vi "Facade.vi"(0 "Data In":T5, 2 "Display State In":T3, 3 "Container State":T4) -> (6 "Data Out":T5, 7 "Display State Out":T3, 8 "Action":T2)   [LabVIEW 2014, in "Mux XControl.xctl"]
uses:
  Mux XControl.xctl
  <vilib>/_xctls/Action.ctl
  <vilib>/_xctls/XControlSupport.lvlib
  <vilib>/_xctls/Container State.ctl
  Data.ctl
  State.ctl
  ChannelType.ctl
panel:
  in  "Channels":T1
  in  "path to image file":path
  out "CtlBckgrnd":picture
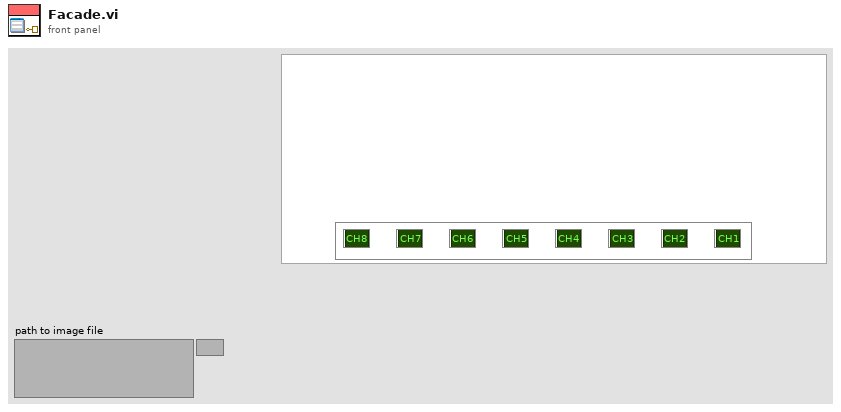
[diagram p1: front panel]
types:
  T1 = cluster{"Ch1":cluster{"StartPoint":cluster{"x":i16, "y":i16}, "RailPoint1":cluster{"x":i16, "y":i16}, "Ch1":bool}, "Ch2":cluster{"StartPoint":cluster{"x":i16, "y":i16}, "RailPoint1":cluster{"x":i16, "y":i16}, "Ch1":bool}, "Ch3":cluster{"StartPoint":cluster{"x":i16, "y":i16}, "RailPoint1":cluster{"x":i16, "y":i16}, "Ch1":bool}, "Ch4":cluster{"StartPoint":cluster{"x":i16, "y":i16}, "RailPoint1":cluster{"x":i16, "y":i16}, "Ch1":bool}, "Ch5":cluster{"StartPoint":cluster{"x":i16, "y":i16}, "RailPoint1":cluster{"x":i16, "y":i16}, "Ch1":bool}, "Ch6":cluster{"StartPoint":cluster{"x":i16, "y":i16}, "RailPoint1":cluster{"x":i16, "y":i16}, "Ch1":bool}, "Ch7":cluster{"StartPoint":cluster{"x":i16, "y":i16}, "RailPoint1":cluster{"x":i16, "y":i16}, "Ch1":bool}, "Ch8":cluster{"StartPoint":cluster{"x":i16, "y":i16}, "RailPoint1":cluster{"x":i16, "y":i16}, "Ch1":bool}}
  T2 = typedef "XControlSupport.lvlib/Action.ctl" = cluster{"Data Changed?":bool, "State Changed?":bool, "Action Name":string}
  T3 = typedef "Mux XControl.xctl/State.ctl" = cluster{"Numeric":dbl}
  T4 = typedef "XControlSupport.lvlib/Container State.ctl" = cluster{"Indicator?":bool, "Run Mode?":bool, " Refnum":refnum<vi>}
  T5 = typedef "Mux XControl.xctl/Data.ctl" = cluster{"From Ch":T6, "Into Ch":T6}
  T6 = typedef "Mux XControl.xctl/ChannelType.ctl" = enum16{"Ch1", "Ch2", "Ch3", "Ch4", "Ch5", "Ch6", "Ch7", "Ch8", "MuxOut"}
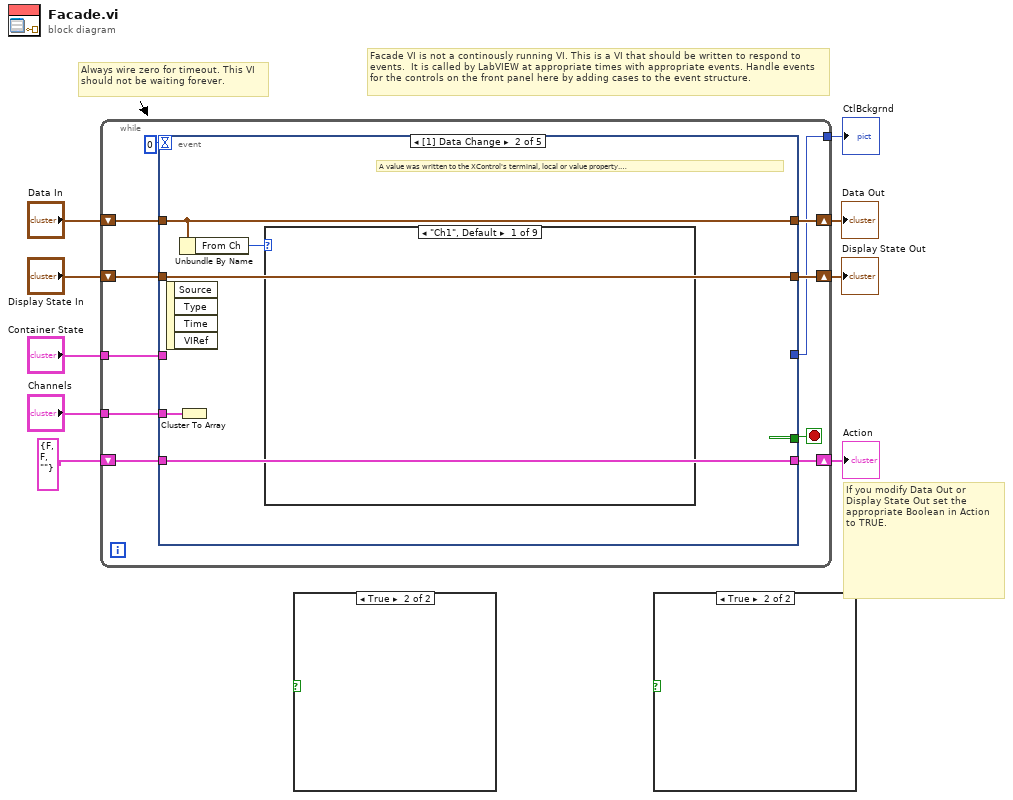
[diagram p0: block diagram]
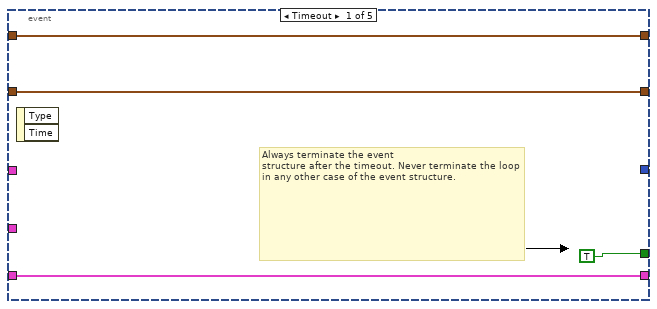
[diagram p4: hidden frame]
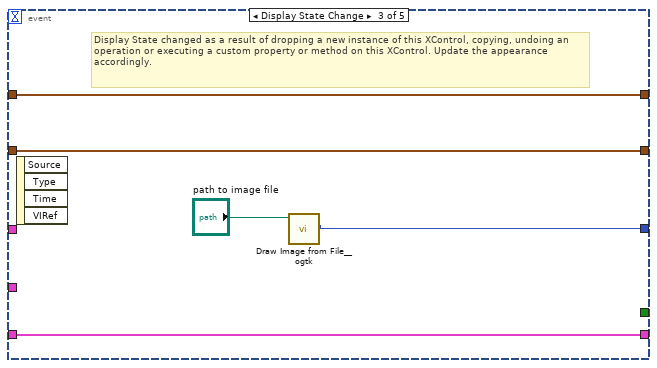
[diagram p13: hidden frame]
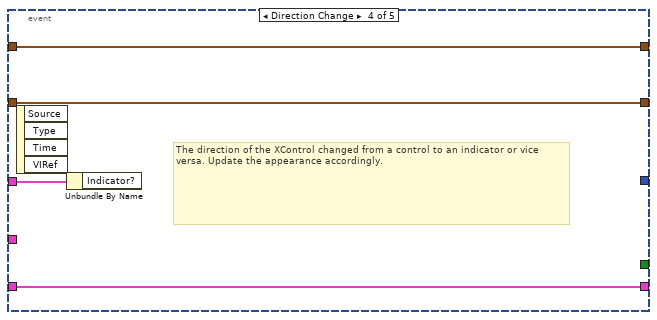
[diagram p14: hidden frame]
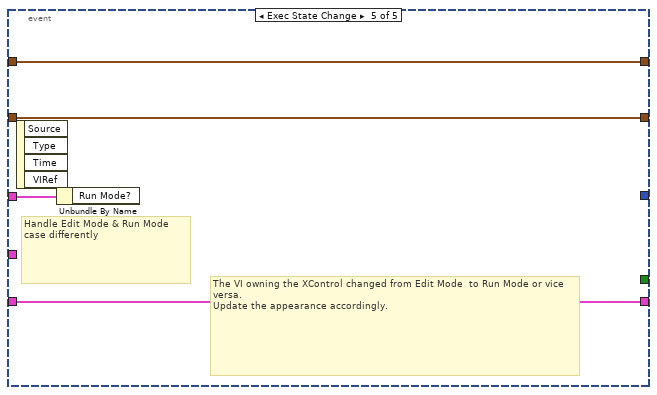
[diagram p15: hidden frame]
diagram:
  # "Always wire zero for timeout. This VI should not be waiting forever."
  # "Facade VI is not a continously running VI. This is a VI that should be written to respond to events.  It is called by LabVIEW at appropriate times with appropriate events. Handle events for the controls on the front panel here by adding cases to the event structure."
  # "If you modify Data Out or\nDisplay State Out set the\nappropriate Boolean in Action\nto TRUE."
  n1 = while {
    shift-right: [w19] -> w6
    shift-left: "Display State In" -> [w20]
    tunnel: "Container State" -> [w16]
    shift-right: [w14] -> w9
    shift-left: "Data In" -> [w15]
    shift-right: [w12] -> w4
    shift-left: T2 {"Data Changed?"=FALSE, "State Changed?"=FALSE, "Action Name"=""} ("Action") -> [w13]
    tunnel: "Channels" -> [w11]
    tunnel: [w10] -> w1
    stop <- w18 stop-if-true
    n2 = event shown="[1] Data Change" {
      selector: _ -> [_ _ _ _ _]
      dyn-events: _ -> [_ _ _ _ _]
      timeout: 0 -> [_ _ _ _ _]
      tunnel: w20 -> [w22 w29 w34 w37 w41]
      tunnel: [w22 w29 w34 w37 w41] -> w19
      tunnel: [TRUE _ _ _ _] -> w18
      tunnel: w16 -> [_ _ _ w38 w42]
      tunnel: w15 -> [w21 w27 w33 w36 w40]
      tunnel: [w21 w27 w33 w36 w40] -> w14
      tunnel: [w23 w28 w32 w35 w39] -> w12
      tunnel: w13 -> [w23 w28 w32 w35 w39]
      tunnel: w11 -> [_ w26 _ _ _]
      tunnel: [_ _ w30 _ _] -> w10
      event Timeout {
        # "Always terminate the event\nstructure after the timeout. Never terminate the loop in any other case of the event structure."
        n3 = event-data() -> ()  [unwired: 1 in, 2 out]
      }
      event Data Change {
        # "A value was written to the XControl's terminal, local or value property.\nUpdate the appearance in response to data change."
        n4 = event-data() -> ()  [unwired: 1 in, 4 out]
        n5 = Cluster To Array(cluster=w26) -> ()  [unwired: 1 out]
        n6 = Unbundle By Name(w27) -> ("From Ch"=w25:T6)
        n7 = case shown="\"Ch1\", Default" w25 {
          frame "Ch1", Default {
          }
          frame "Ch2" {
          }
          frame "Ch3" {
          }
          frame "Ch4" {
          }
          frame "Ch5" {
          }
          frame "Ch6" {
          }
          frame "Ch7" {
          }
          frame "Ch8" {
          }
          frame "MuxOut" {
          }
        }
      }
      event Display State Change {
        # "Display State changed as a result of dropping a new instance of this XControl, copying, undoing an operation or executing a custom property or method on this XControl. Update the appearance accordingly."
        n8 = event-data() -> ()  [unwired: 1 in, 4 out]
        n9 = call <userlib>:"Draw Image from File__ogtk.vi"("path to image file"="path to image file") -> ("new picture"=w30:picture)  [unwired: 7 in, 3 out]
      }
      event Direction Change {
        # "The direction of the XControl changed from a control to an indicator or vice versa. Update the appearance accordingly."
        n10 = event-data() -> ()  [unwired: 1 in, 4 out]
        n11 = Unbundle By Name(w38) -> ()  [unwired: 1 out]
      }
      event Exec State Change {
        # "The VI owning the XControl changed from Edit Mode  to Run Mode or vice versa.\nUpdate the appearance accordingly."
        # "Handle Edit Mode & Run Mode\ncase differently"
        n12 = event-data() -> ()  [unwired: 1 in, 4 out]
        n13 = Unbundle By Name(w42) -> ()  [unwired: 1 out]
      }
    }
  }
  "Display State Out" <- w6
  "Data Out" <- w9
  "Action" <- w4
  "CtlBckgrnd" <- w1
  n14 = case shown="True" {
    selector: _ -> [_ _]
    frame False {
    }
    frame True {
    }
  }
  n15 = case shown="True" {
    selector: _ -> [_ _]
    frame False {
    }
    frame True {
    }
  }
